vi "UMLEditor_IniFilePath.vi"(0 "SetPath(if not empty)":path=path "", 2 "error in (no error)":errorcluster) -> (14 "Get Path":path, 16 "error out":errorcluster)   [LabVIEW 2016]
doc: "This VI is used to manage system paths.\n\nName: The name of the path to be set or retrieved. The default Name is Home.\n\nPath In: Used to specify the path for Set Path method.\n\nPath Out: Returns the path for Get Path method.\n\nerror out: Returns error info if appropriate.\n\nMethod: {Get Path, Set Path, Delete Path, Clear All Paths}\n\nAuthor: SPCase\nCopyright 2003 VI Engineering, Inc.\n\nCurrent Revision: 12\nVSS Version: 2"
uses:
  <vilib>/Utility/config.llb/Write Key (Path).vi
  <vilib>/Utility/config.llb/Read Key (Path).vi
  <vilib>/Utility/config.llb/NI_LVConfig.lvlib
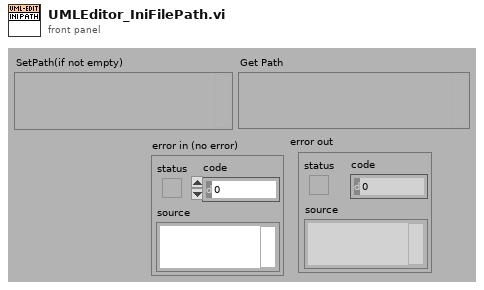
[diagram p1: front panel]
types:
  T1 = typedef "NI_LVConfig.lvlib/Config Data RefNum.ctl" = refnum<k1>
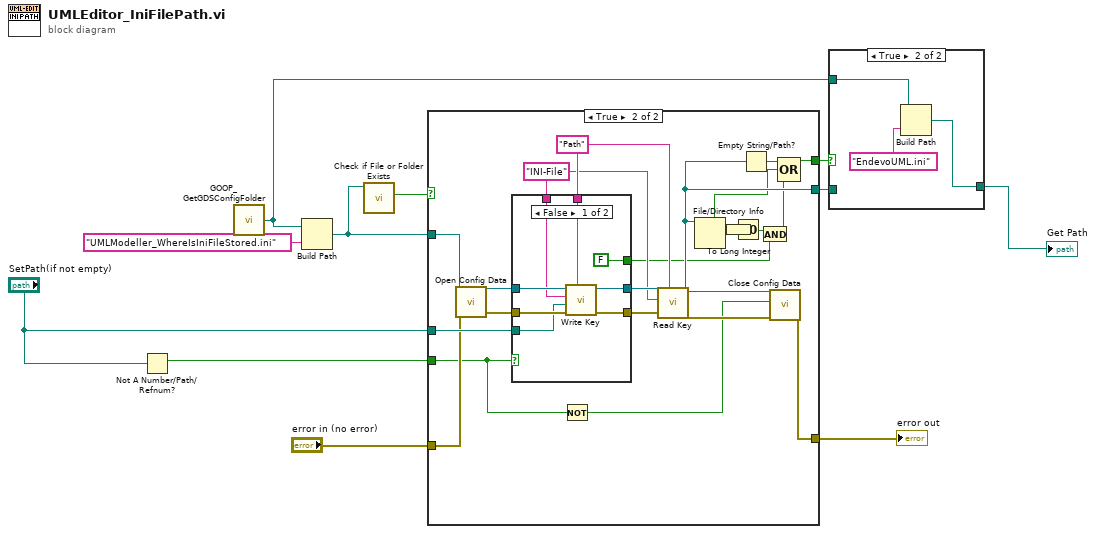
[diagram p0: block diagram]
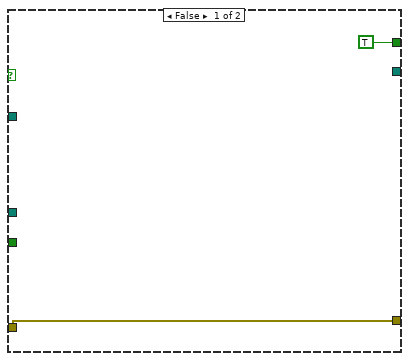
[diagram p2: hidden frame]
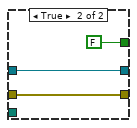
[diagram p3: hidden frame]
diagram:
  n1 = Not A Number/Path/Refnum?(number/path/refnum="SetPath(if not empty)") -> (NaN/Path/Refnum?=w7:bool)
  n2 = call <resource>:"GOOP_GetGDSConfigFolder.vi"() -> ("GDSFolderPath"=w3:path)
  n3 = Build Path(base path=w3, name or relative path="UMLModeller_WhereIsIniFileStored.ini") -> (appended path=w2:path)
  n4 = call <vilib>:"Check if File or Folder Exists.vi"("path"=w2) -> ("file or folder exists?"=w1:bool)  [unwired: 8 in, 2 out]
  n5 = case shown="True" w1 {
    tunnel: "SetPath(if not empty)" -> [_ w34]
    tunnel: "error in (no error)" -> [w12 w31]
    tunnel: [w12 w26] -> w8
    tunnel: w7 -> [_ w25]
    tunnel: [_ w23] -> w5
    tunnel: [TRUE w19] -> w4
    tunnel: w2 -> [_ w14]
    frame False {
    }
    frame True {
      w29 = "INI-File" ("section")
      w30 = "Path" ("section")
      n6 = call <vilib>:"Open Config Data.vi"("error in (no error)"=w31, "configuration file path"=w14) -> ("error out"=w36:errorcluster, "refnum"=w35:T1)  [unwired: 7 in, 1 out]
      n7 = case shown="False" w25 {
        tunnel: w36 -> [w44 w46]
        tunnel: w35 -> [w43 w47]
        tunnel: w34 -> [w42 _]
        tunnel: [w41 w47] -> w33
        tunnel: [w40 w46] -> w32
        tunnel: w29 -> [w39 _]
        tunnel: w30 -> [w38 _]
        tunnel: [FALSE FALSE] -> w16
        frame False {
          n8 = call-poly <vilib>:"Write Key.vi"("section"=w38, "error in (no error)"=w44, "value"=w42, "key"=w39, "refnum"=w43) -> ("error out"=w40:errorcluster, "refnum out"=w41:T1)  [unwired: 5 out]
        }
        frame True {
        }
      }
      n9 = Not(x=w25) -> (.not. x?=w24:bool)
      n10 = call-poly <vilib>:"Read Key.vi"("section"=w30, "error in (no error)"=w32, "key"=w29, "refnum"=w33) -> ("error out"=w27:errorcluster, "value"=w23:path, "refnum out"=w28:T1)  [unwired: 1 in, 4 out]
      n11 = File/Directory Info(path=w23) -> (directory=w20:bool, size=w15:i64)  [unwired: 1 in, 5 out]
      n12 = To Long Integer(number=w15) -> (32bit integer=w21:i32)
      n13 = Equal To 0?(x=w21) -> (x = 0?=w17:bool)
      n14 = Empty String/Path?(string/path=w23) -> (empty?=w22:bool)
      n15 = And(x=w17, y=w16) -> (x .and. y?=w18:bool)
      n16 = call <vilib>:"Close Config Data.vi"("error in (no error)"=w27, "write file if changed (T)"=w24, "refnum"=w28) -> ("error out"=w26:errorcluster)  [unwired: 8 out]
      n17 = Compound Arithmetic op=OR(w22, w20, w18) -> (w19:bool)
    }
  }
  "error out" <- w8
  n18 = case shown="True" w4 {
    tunnel: [w48 w50] -> w6
    tunnel: w5 -> [w48 _]
    tunnel: w3 -> [_ w49]
    frame False {
    }
    frame True {
      n19 = Build Path(base path=w49, name or relative path="EndevoUML.ini" ("string")) -> (appended path=w50:path)
    }
  }
  "Get Path" <- w6
